vi "5492_YawDecision.vi"(10 "Yaw Goallll":dbl, 11 "Parsed Yaw":dbl) -> (3 "Right???":bool)   [LabVIEW 2016]
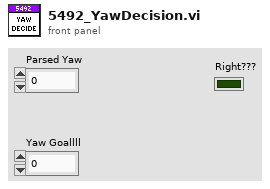
[diagram p1: front panel]
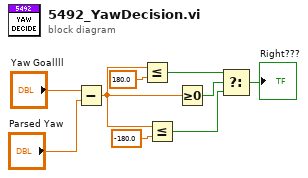
[diagram p0: block diagram]
diagram:
  n1 = Subtract(x="Yaw Goallll", y="Parsed Yaw") -> (x-y=w4:dbl)
  n2 = Less Or Equal?(x=w4, y=180.0) -> (x <= y?=w6:bool)
  n3 = Less Or Equal?(x=w4, y=-180.0) -> (x <= y?=w2:bool)
  n4 = Greater Or Equal To 0?(x=w4) -> (x >= 0?=w7:bool)
  n5 = Select(t=w6, s=w7, f=w2) -> (s? t:f=→"Right???":bool)
